vi "GUI.vi"() -> ()   [LabVIEW 2021]
uses:
  Data.ctl
  Case.ctl
  <vilib>/httpClient/ClientHandle.ctl
  <vilib>/JDP Science/JSONtext/Next JSON Value.vi
  <vilib>/JDP Science/JSONtext/String Subset.vi
  <vilib>/JDP Science/JSONtext/Parsing/Advance past next JSON Value (inlined COPY).vi
  <vilib>/JDP Science/JSONtext/Parsing/Advance past whitespace.vi
  <vilib>/JDP Science/JSONtext/Parsing/Advance past String.vi
  <vilib>/JDP Science/JSONtext/Parsing/Advance past Number.vi
  <vilib>/JDP Science/JSONtext/Parsing/Advance past Line Ending.vi
  <vilib>/JDP Science/JSONtext/Parsing/Parse Full Path or Item Name.vi
  <vilib>/JDP Science/JSONtext/Parsing/Advance past Array.vi
  <vilib>/JDP Science/JSONtext/Parsing/Advance past Object.vi
  <vilib>/JDP Science/JSONtext/support/Error Cluster From Code.vi
  <vilib>/JDP Science/JSONtext/Offset/Find Item Locations by Path.vi
  <vilib>/httpClient/POSTBuffer.vi
  <vilib>/httpClient/LabVIEWHTTPClient.lvlib
  <vilib>/JDP Science/JSONtext/JSONtext.lvlib
panel:
  out "Voltage":dbl
  out "error out":errorcluster
  out "While":bool caption="3"
  in  "IP Address":string
  out "Red":bool caption="2"
  out "Yellow":bool caption="1"
  out "Green":bool caption="0"
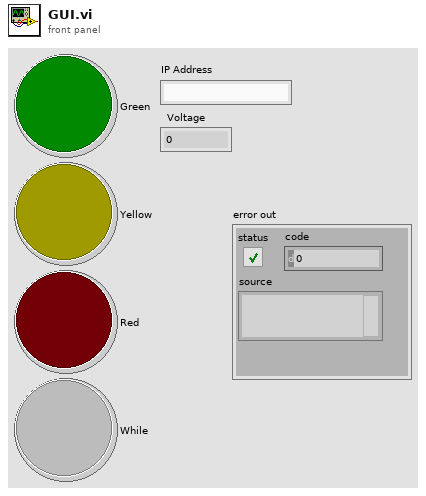
[diagram p1: front panel]
types:
  T1 = typedef "Data.ctl" = cluster{"Enum":T2, "Data":variant}
  T2 = typedef "Case.ctl" = enum16{"Initialize", "LightStatus", "Parsing light", "Change light", "Close", "Change ip"}
  T3 = typedef "LabVIEWHTTPClient.lvlib/ClientHandle.ctl" = refnum<k1>
  T4 = cluster{"IP Address":string, "timeout (10000)":i32, "client":T3, "body":string, "url":string}
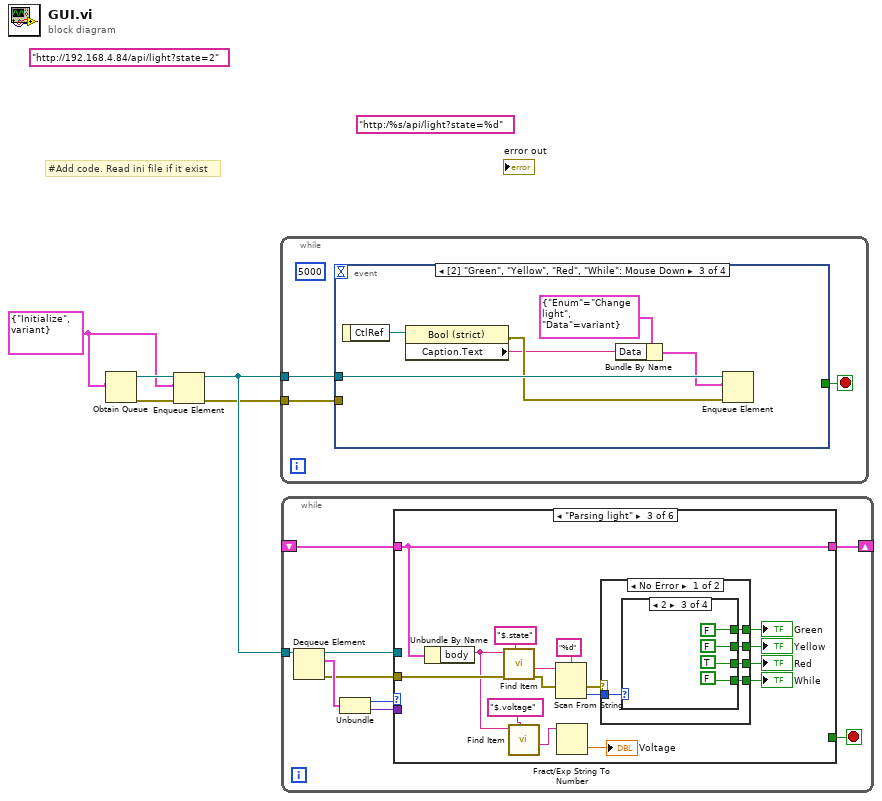
[diagram p0: block diagram]
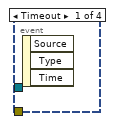
[diagram p2: hidden frame]
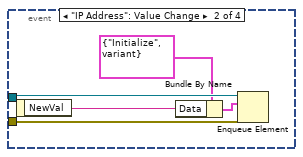
[diagram p3: hidden frame]
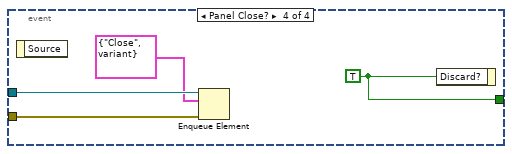
[diagram p4: hidden frame]
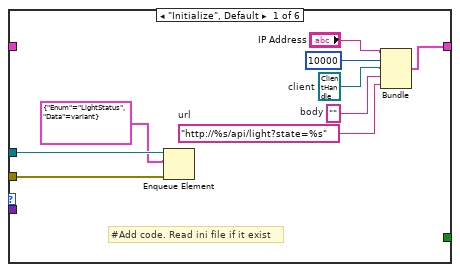
[diagram p5: hidden frame]
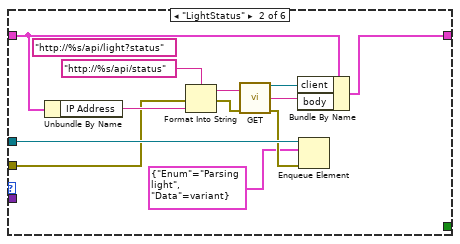
[diagram p6: hidden frame]
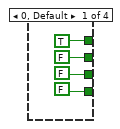
[diagram p7: hidden frame]
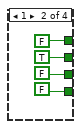
[diagram p8: hidden frame]
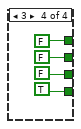
[diagram p9: hidden frame]
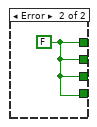
[diagram p10: hidden frame]
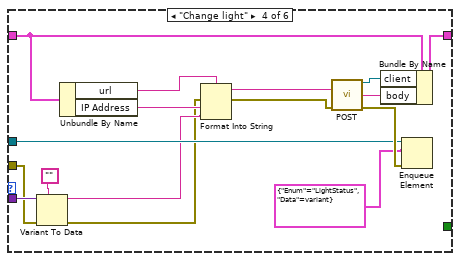
[diagram p11: hidden frame]
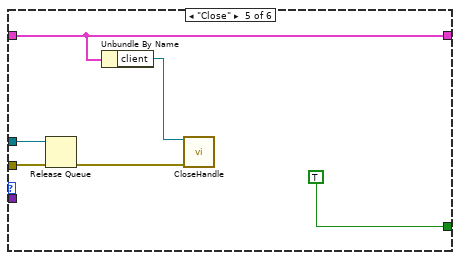
[diagram p12: hidden frame]
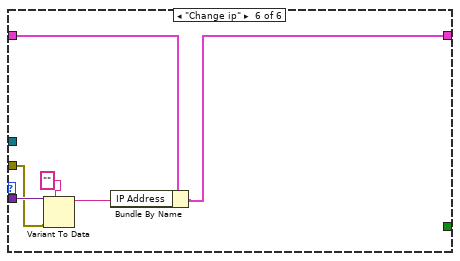
[diagram p13: hidden frame]
diagram:
  w4 = T1 {"Enum"=enum."Initialize", "Data"=variant} ("Message")
  (unwired) "http:/%s/api/light?state=%d" ("url")
  (unwired) "http://192.168.4.84/api/light?state=2" ("url")
  # "#Add code. Read ini file if it exist"
  n1 = Obtain Queue(element data type=w4) -> (queue out=w5:refnum<queue>, error out=w3:errorcluster)  [unwired: 4 in, 1 out]
  n2 = Enqueue Element(queue=w5, element=w4, error in (no error)=w3) -> (queue out=w2:refnum<queue>, error out=w1:errorcluster)  [unwired: 1 in, 1 out]
  n3 = while {
    tunnel: w2 -> [w7]
    tunnel: w1 -> [w6]
    stop <- w8 stop-if-true
    (unwired) 5000
    n4 = event shown="[2] \"Green\", \"Yellow\", \"Red\", \"While\": Mouse Down" {
      selector: _ -> [_ _ _ _]
      dyn-events: _ -> [_ _ _ _]
      timeout: _ -> [_ _ _ _]
      tunnel: [_ _ _ w23] -> w8
      tunnel: w7 -> [_ w12 w19 w22]
      tunnel: w6 -> [_ w13 _ w21]
      event Timeout {
        n5 = event-data() -> ()  [unwired: 1 in, 3 out]
      }
      event "IP Address": Value Change {
        n6 = event-data() -> ("NewVal"=w9:string)  [unwired: 1 in]
        n7 = Bundle By Name(cluster=T1 {"Enum"=enum."Initialize", "Data"=variant} ("Message"), "Data"=w9) -> (w10:T1)
        n8 = Enqueue Element(queue=w12, element=w10, error in (no error)=w13) -> ()  [unwired: 1 in, 3 out]
      }
      event "Green", "Yellow", "Red", "While": Mouse Down {
        n9 = event-data() -> ("CtlRef"=w18:refnum<vi>)  [unwired: 1 in]
        n10 = property class="Bool (strict)"(reference=w18) -> (error out=w17:errorcluster, "Caption.Text"=w15:string)  [unwired: 1 in, 1 out]
        n11 = Bundle By Name(cluster=T1 {"Enum"=enum."Change light", "Data"=variant} ("Message"), "Data"=w15) -> (w14:T1)
        n12 = Enqueue Element(queue=w19, element=w14, error in (no error)=w17) -> ()  [unwired: 1 in, 3 out]
      }
      event Panel Close? {
        w23 = TRUE ("Discard?")
        n13 = event-data() -> ()  [unwired: 1 in, 1 out]
        n14 = Enqueue Element(queue=w22, element=T1 {"Enum"=enum."Close", "Data"=variant} ("Message"), error in (no error)=w21) -> ()  [unwired: 1 in, 3 out]
        n15 = event-data("Discard?"=w23) -> ()  [unwired: 1 in, 1 out]
      }
    }
  }
  n16 = while {
    tunnel: w2 -> [w32]
    shift-right: [w24] -> _
    shift-left: _ -> [w25]
    stop <- w27 stop-if-true
    n17 = Dequeue Element(queue=w32) -> (queue out=w29:refnum<queue>, element=w31:T1, error out=w28:errorcluster)  [unwired: 2 in, 1 out]
    n18 = Unbundle(w31) -> ("Enum"=w30:T2, "Data"=w26:variant)
    n19 = case shown="\"Parsing light\"" w30 {
      tunnel: w29 -> [w40 w53 _ w105 w113 _]
      tunnel: w28 -> [w39 w43 w68 w93 w112 w114]
      tunnel: [_ _ _ _ TRUE _] -> w27
      tunnel: w26 -> [_ _ _ w99 _ w119]
      tunnel: w25 -> [_ w51 w69 w107 w110 w117]
      tunnel: [w41 w48 w69 w102 w110 w115] -> w24
      frame "Initialize", Default {
        w33 = "http://%s/api/light?state=%s"  # url
        w35 = ""  # body
        w36 = T3 refnum  # client
        # "#Add code. Read ini file if it exist"
        n20 = Enqueue Element(queue=w40, element=T1 {"Enum"=enum."LightStatus", "Data"=variant} ("Message"), error in (no error)=w39) -> ()  [unwired: 1 in, 3 out]
        n21 = Bundle("IP Address"="IP Address", "timeout (10000)"=10000, "client"=w36, "body"=w35, "url"=w33) -> (w41:T4)  [unwired: 1 in]
      }
      frame "LightStatus" {
        (unwired) "http://%s/api/light?status" ("url")
        n22 = Unbundle By Name(w51) -> ("IP Address"=w50:string)
        n23 = Format Into String(format string="http://%s/api/status" ("url"), error in=w43, w50) -> (resulting string=w52:string, error out=w44:errorcluster)  [unwired: 1 in]
        n24 = call <vilib>:"GET.vi"("url"=w52, "error in (no error)"=w44) -> ("client handle out"=w47:T3, "body"=w46:string, "error out"=w49:errorcluster)  [unwired: 10 in, 1 out]
        n25 = Bundle By Name(cluster=w51, "client"=w47, "body"=w46) -> (w48:T4)
        n26 = Enqueue Element(queue=w53, element=T1 {"Enum"=enum."Parsing light", "Data"=variant} ("Message"), error in (no error)=w49) -> ()  [unwired: 1 in, 3 out]
      }
      frame "Parsing light" {
        n27 = Unbundle By Name(w69) -> ("body"=w57:string)
        n28 = call <vilib>:"Find Item.vi"("$Path or Item Name"="$.state", "error in (no error)"=w68, "JSON"=w57) -> ("error out"=w65:errorcluster, "<JSON>"=w66:string)  [unwired: 5 in, 2 out]
        n29 = call <vilib>:"Find Item.vi"("$Path or Item Name"="$.voltage", "JSON"=w57) -> ("<JSON>"=w55:string)  [unwired: 6 in, 3 out]
        n30 = Scan From String(format string="%d" ("$Path or Item Name"), input string=w66, error in=w65) -> (error out=w64:errorcluster, output 1=w63:i32)  [unwired: 2 in, 2 out]
        n31 = Fract/Exp String To Number(string=w55) -> (number=→"Voltage":dbl)  [unwired: 3 in, 1 out]
        n32 = case shown="No Error" w64 {
          tunnel: w63 -> [w74 _]
          tunnel: [w73 w91] -> w61
          tunnel: [w72 w91] -> w60
          tunnel: [w71 w91] -> w59
          tunnel: [w70 w91] -> w58
          frame No Error {
            n33 = case shown="2" w74 {
              tunnel: [TRUE FALSE FALSE FALSE] -> w73
              tunnel: [FALSE TRUE FALSE FALSE] -> w72
              tunnel: [FALSE FALSE TRUE FALSE] -> w71
              tunnel: [FALSE FALSE FALSE TRUE] -> w70
              frame 0, Default {
              }
              frame 1 {
              }
              frame 2 {
              }
              frame 3 {
              }
            }
          }
          frame Error {
            w91 = FALSE
          }
        }
        "Green" <- w61
        "Yellow" <- w60
        "Red" <- w59
        "While" <- w58
      }
      frame "Change light" {
        n34 = Variant To Data(error in=w93, type="", Variant=w99) -> (data=w97:string, error out=w94:errorcluster)
        n35 = Unbundle By Name(w107) -> ("url"=w92:string, "IP Address"=w95:string)
        n36 = Format Into String(format string=w92, error in=w94, w95, w97) -> (resulting string=w103:string, error out=w96:errorcluster)  [unwired: 1 in]
        n37 = call-poly <vilib>:"POST.vi"("url"=w103, "error in (no error)"=w96) -> ("client handle out"=w100:T3, "body"=w101:string, "error out"=w106:errorcluster)  [unwired: 10 in, 1 out]
        n38 = Bundle By Name(cluster=w107, "client"=w100, "body"=w101) -> (w102:T4)
        n39 = Enqueue Element(queue=w105, element=T1 {"Enum"=enum."LightStatus", "Data"=variant} ("Message"), error in (no error)=w106) -> ()  [unwired: 1 in, 3 out]
      }
      frame "Close" {
        n40 = Release Queue(queue=w113, error in (no error)=w112) -> (error out=w108:errorcluster)  [unwired: 1 in, 2 out]
        n41 = Unbundle By Name(w110) -> ("client"=w109:T3)
        n42 = call <vilib>:"CloseHandle.vi"("client handle"=w109, "error in (no error)"=w108) -> ()  [unwired: 13 in, 1 out]
      }
      frame "Change ip" {
        n43 = Variant To Data(error in=w114, type="" ("url"), Variant=w119) -> (data=w116:string)  [unwired: 1 out]
        n44 = Bundle By Name(cluster=w117, "IP Address"=w116) -> (w115:T4)
      }
    }
  }
